vi "myRIO_BRig_Host_formatData_test2_p2.vi"(7 "input_headers":string[](array[string]), 8 "input_error":errorcluster, 9 "input_Iexist":bool, 10 "input_filePath":path, 11 "input_hdl_Workbooks":refnum<k7>) -> (0 "output_error":errorcluster, 2 "output_newFilePath":path, 3 "output_hdl_Worksbooks":refnum<k7>)   [LabVIEW 2014]
uses:
  <vilib>/Utility/file.llb/Read From Spreadsheet File (I64).vi
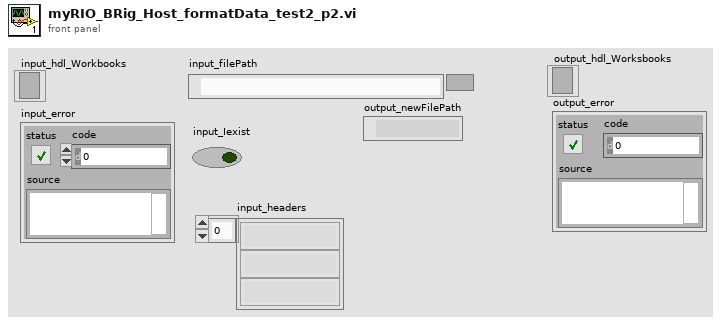
[diagram p1: front panel]
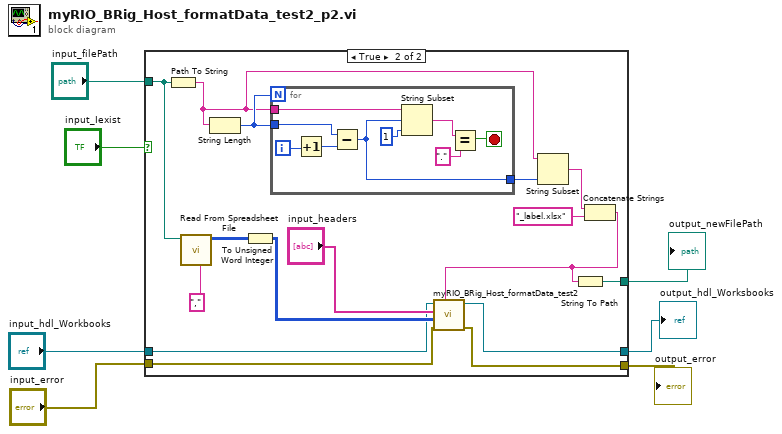
[diagram p0: block diagram]
diagram:
  n1 = case shown="True" "input_Iexist" {
    tunnel: "input_hdl_Workbooks" -> [w9 w16]
    tunnel: "input_error" -> [w8 w15]
    tunnel: [w9 w13] -> w3
    tunnel: [w8 w14] -> w2
    tunnel: "input_filePath" -> [_ w12]
    tunnel: [_ w10] -> w1
    frame False {
    }
    frame True {
      n2 = Path To String(path=w12) -> (string=w23:string)
      n3 = call-poly <vilib>:"Read From Spreadsheet File.vi"("delimiter (\\t)"="," ("delimiter (\\t)"), "file path (dialog if empty)"=w12) -> ("all rows"=w19:i64[][])  [unwired: 5 in, 4 out]
      n4 = String Length(string=w23) -> (length=w25:i32)
      n5 = To Unsigned Word Integer(number=w19) -> (unsigned 16bit integer=w18:u16[][])
      n6 = for {
        N: w25 -> [_]
        tunnel: w25 -> [w32]
        tunnel: w23 -> [w31]
        tunnel: [w26] -> w24
        i -> [w34]
        stop <- w27 stop-if-true
        n7 = Increment(x=w34) -> (x+1=w33:i32)
        n8 = Subtract(x=w32, y=w33) -> (x-y=w26:i32)
        n9 = String Subset(string=w31, offset (0)=w26, length (rest)=1 ("length (rest)")) -> (substring=w29:string)
        n10 = Equal?(x=w29, y=".") -> (x = y?=w27:bool)
      }
      n11 = String Subset(string=w23, length (rest)=w24) -> (substring=w22:string)  [unwired: 1 in]
      n12 = Concatenate Strings(w22, "_label.xlsx" ("string")) -> (w11:string)
      n13 = call "myRIO_BRig_Host_formatData_test2.vi"("input_filePath"=w11, "input_error"=w15, "input_data"=w18, "input_headers"="input_headers", "input_hdl_Workbooks"=w16) -> ("output_error"=w14:errorcluster, "output_hdl_Worksbooks"=w13:refnum<k7>)  [unwired: 5 in]
      n14 = String To Path(string=w11) -> (path=w10:path)
    }
  }
  "output_hdl_Worksbooks" <- w3
  "output_error" <- w2
  "output_newFilePath" <- w1
